vi "DAQ_AcquireInterferogram.vi"(9 "Sampling rate":dbl, 10 "Time per acquisiton (s)":dbl) -> (3 "Output V-d array":dbl[][](array[numeric]))   [LabVIEW 2021]
panel:
  out "Acquisition cycle":dbl[][](graph)
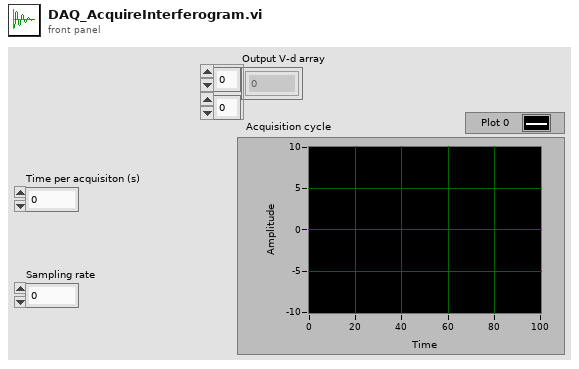
[diagram p1: front panel]
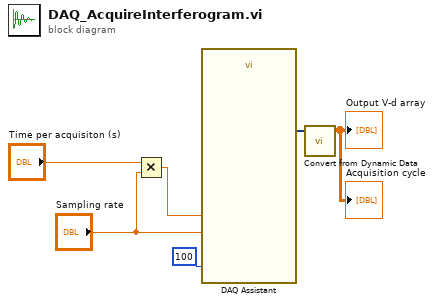
[diagram p0: block diagram]
diagram:
  n1 = Multiply(x="Time per acquisiton (s)", y="Sampling rate") -> (x*y=w5:dbl)
  n2 = call "DAQ Assistant"("rate"="Sampling rate", "number of samples"=w5, "timeout (s)"=100) -> ("data"=w6:dynamicdata)  [unwired: 14 in, 2 out]
  n3 = call "Convert from Dynamic Data"("Dynamic Data Type"=w6) -> ("Array"=→"Output V-d array" →"Acquisition cycle":dbl[][])  [unwired: 3 in]
